vi "Query Reading Buffer Storage Status.vi"(8 "error in (no error)":errorcluster, 10 "Reading Buffer (smua.nvbuffer1)":string="smua.nvbuffer1", 11 "VISA resource name":refnum<visa-resource-name>) -> (0 "error out":errorcluster, 1 "Data Length":i32, 2 "Buffer Size":i32, 3 "VISA resource name out":refnum<visa-resource-name>, 5 "Base Time":timestamp)   [LabVIEW 2015, in "Keithley 2600 Series.lvlib"]
doc: "Returns the capacity of the buffer and the number of readings stored in the buffer."
uses:
  Keithley 2600 Series.lvlib
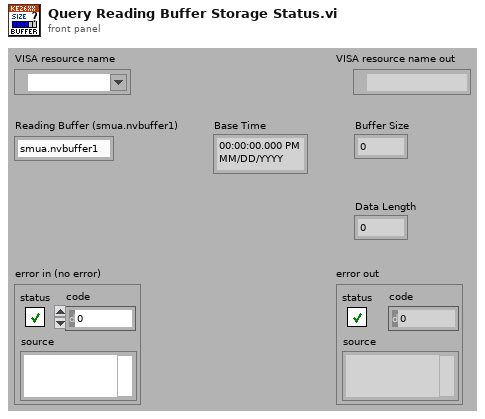
[diagram p1: front panel]
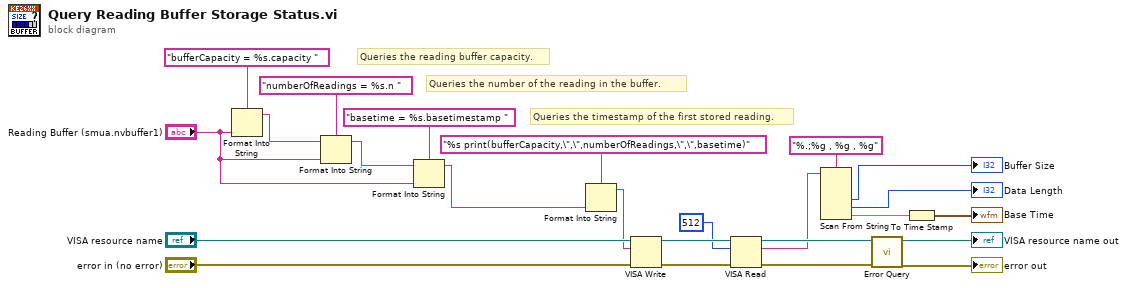
[diagram p0: block diagram]
diagram:
  # "Queries the number of the reading in the buffer."
  # "Queries the reading buffer capacity."
  # "Queries the timestamp of the first stored reading."
  n1 = Format Into String(format string="bufferCapacity = %s.capacity ", "Reading Buffer (smua.nvbuffer1)") -> (resulting string=w23:string)  [unwired: 2 in, 1 out]
  n2 = Format Into String(format string="numberOfReadings = %s.n ", initial string=w23, "Reading Buffer (smua.nvbuffer1)") -> (resulting string=w20:string)  [unwired: 1 in, 1 out]
  n3 = Format Into String(format string="basetime = %s.basetimestamp ", initial string=w20, "Reading Buffer (smua.nvbuffer1)") -> (resulting string=w14:string)  [unwired: 1 in, 1 out]
  n4 = Format Into String(format string="%s print(bufferCapacity,\",\",numberOfReadings,\",\",basetime)", w14) -> (resulting string=w12:string)  [unwired: 2 in, 1 out]
  n5 = VISA Write(VISA resource name="VISA resource name", write buffer=w12, error in (no error)="error in (no error)") -> (VISA resource name out=w11:refnum<visa-resource-name>, error out=w9:errorcluster)  [unwired: 1 out]
  n6 = VISA Read(VISA resource name=w11, byte count=u32 512, error in (no error)=w9) -> (VISA resource name out=w10:refnum<visa-resource-name>, read buffer=w6:string, error out=w8:errorcluster)  [unwired: 1 out]
  n7 = Scan From String(format string="%.;%g , %g , %g", input string=w6) -> (output 1=→"Buffer Size":i32, output 2=→"Data Length":i32, output 3=w2:dbl)  [unwired: 5 in, 3 out]
  n8 = call "Error Query.vi"("error in (no error)"=w8, "VISA resource name"=w10) -> ("error out"=→"error out":errorcluster, "VISA resource name out"=→"VISA resource name out":refnum<visa-resource-name>)  [unwired: 6 in, 2 out]
  n9 = To Time Stamp(1:w2) -> (0:→"Base Time":timestamp)
